vi "SVPWMabcSGL.vi"(0 "A":sgl, 1 "SVPWM_SGL":T1={"max"=0.9999695, "Period"=0, "Deadtime"=1}, 5 "B":sgl, 7 "C":sgl, 9 "input valid":bool=TRUE, 12 "enable":bool=TRUE) -> (4 "SwitchPositions":T2, 14 "Sector":u8, 15 "ready for input":bool)   [LabVIEW 2015, in "SVPWM.lvlib"]
uses:
  SVPWM.lvlib
  SwitchPositions.ctl
  SVPWM_SGL.ctl
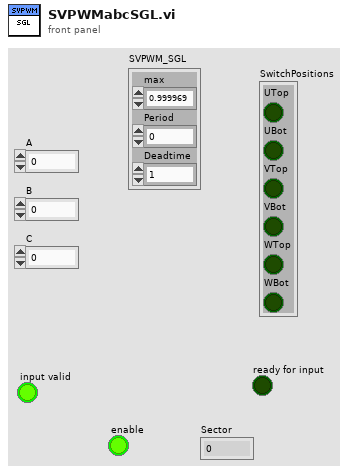
[diagram p1: front panel]
types:
  T1 = typedef "SVPWM.lvlib/SVPWM_SGL.ctl" = cluster{"max":sgl, "Period":u32, "Deadtime":u8}
  T2 = typedef "SVPWM.lvlib/SwitchPositions.ctl" = cluster{"UTop":bool, "UBot":bool, "VTop":bool, "VBot":bool, "WTop":bool, "WBot":bool}
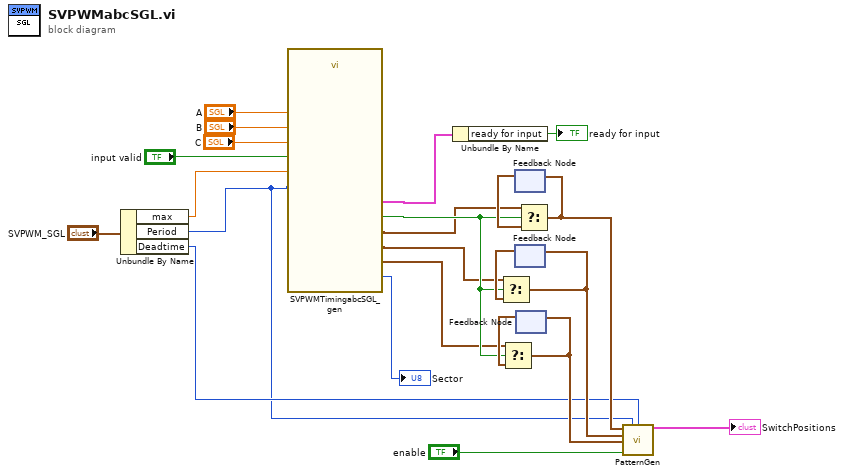
[diagram p0: block diagram]
diagram:
  n1 = Unbundle By Name("SVPWM_SGL") -> ("max"=w5:sgl, "Period"=w4:u32, "Deadtime"=w14:u8)
  n2 = call "SVPWMTimingabcSGL_gen.vi"("C"="C", "A"="A", "B"="B", "Period"=w4, "input valid"="input valid", "max"=w5) -> ("Sector"=→"Sector":u8, "W_timing"=w10:cluster{"ON":u32, "OFF":u32}, "V_Timing"=w11:cluster{"ON":u32, "OFF":u32}, "output valid"=w12:bool, "feedback signals"=w13:cluster{"ready for input":bool}, "U_Timing"=w2:cluster{"ON":u32, "OFF":u32})  [unwired: 4 in]
  n3 = Unbundle By Name(w13) -> ("ready for input"=→"ready for input":bool)
  n4 = feedback #1() -> (w23:cluster{"ON":u32, "OFF":u32})  [unwired: 1 in]
  n5 = feedback #2() -> (w22:cluster{"ON":u32, "OFF":u32})  [unwired: 1 in]
  n6 = Select(t=w10, s=w12, f=w22) -> (s? t:f=w19:cluster{"ON":u32, "OFF":u32})
  n7 = feedback-in #2(w19) -> ()
  n8 = feedback #3() -> (w21:cluster{"ON":u32, "OFF":u32})  [unwired: 1 in]
  n9 = Select(t=w2, s=w12, f=w21) -> (s? t:f=w18:cluster{"ON":u32, "OFF":u32})
  n10 = feedback-in #3(w18) -> ()
  n11 = Select(t=w11, s=w12, f=w23) -> (s? t:f=w20:cluster{"ON":u32, "OFF":u32})
  n12 = feedback-in #1(w20) -> ()
  n13 = call "PatternGen.vi"("U_timing"=w20, "Period"=w4, "Deadtime"=w14, "V_timing"=w19, "W_timing"=w18, "enable"="enable") -> ("SwitchPositions"=→"SwitchPositions":T2)  [unwired: 9 in]
